vi "Take Outline Image.vi"(5 "Outline Width":dbl, 6 "Image Name":string="composite image", 7 "Quality":enum16{"perfect", "high", "medium", "low"}(ring), 8 "error in":errorcluster, 9 "Field of View":cluster{"Size-X(mm)":dbl, "Size-Y(mm)":dbl}, 10 "Image Center":refnum<class "Vec3d Class.lvclass">, 11 "CameraTool in":refnum<class "CameraTool Class.lvclass">) -> (0 "error out":errorcluster, 2 "Physical Image":T1, 3 "CameraTool out":refnum<class "CameraTool Class.lvclass">)   [LabVIEW 2017, in "CameraTool Class.lvclass"]
uses:
  CameraTool Class.lvclass
  Vec3d Class/Vec3d Class.lvclass
  <vilib>/vision/Image Controls.llb/IMAQ Image.ctl
  Utils/Type Definitions/Physical Image.ctl
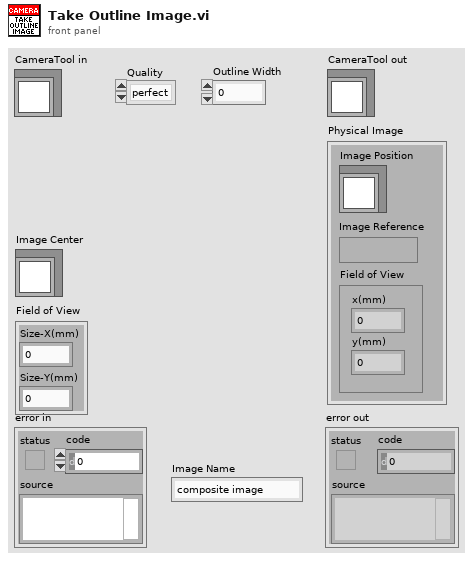
[diagram p1: front panel]
types:
  T1 = typedef "Physical Image.ctl" = cluster{"Image Position":refnum<class "Vec3d Class.lvclass">, "Image Reference":T2, "Field of View":cluster{"x(mm)":dbl, "y(mm)":dbl}}
  T2 = typedef "IMAQ Image.ctl" = refnum<image>
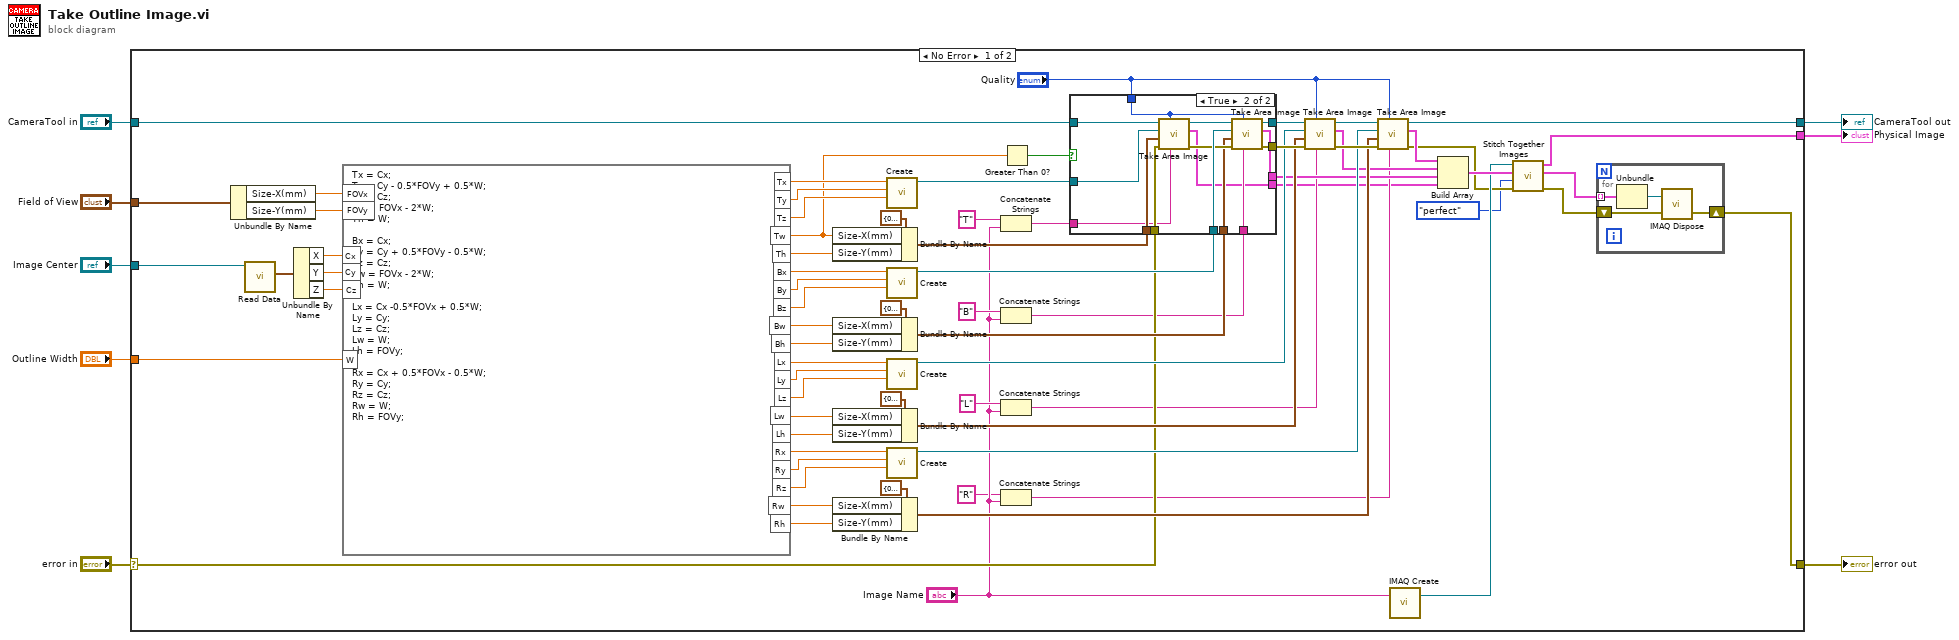
[diagram p0: block diagram]
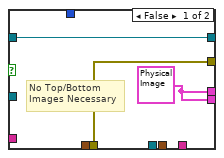
[diagram p2: hidden frame]
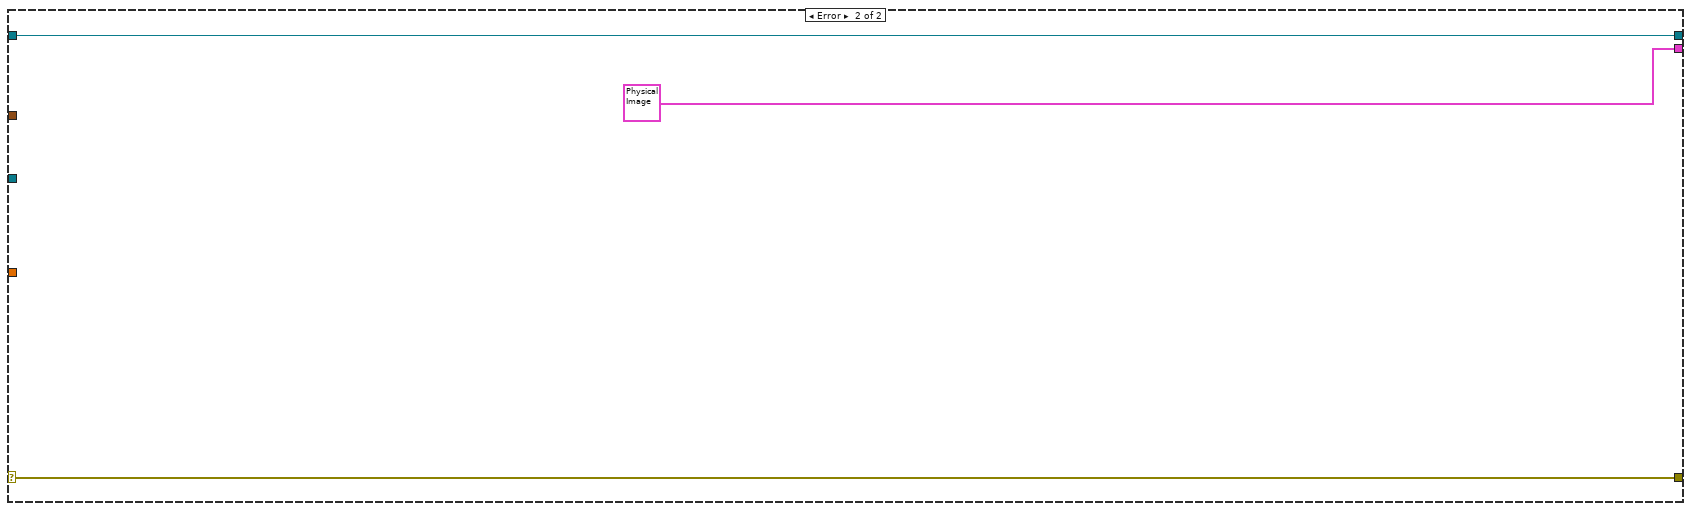
[diagram p3: hidden frame]
diagram:
  n1 = case shown="No Error" "error in" {
    selector: "error in" -> [w33 w104]
    tunnel: [w14 w104] -> w7
    tunnel: [w44 w103] -> w5
    tunnel: "CameraTool in" -> [w47 w103]
    tunnel: "Field of View" -> [w78 _]
    tunnel: "Image Center" -> [w79 _]
    tunnel: [w26 T1 {"Image Position"=refnum, "Image Reference"=refnum, "Field of View"={"x(mm)"=0.0, "y(mm)"=0.0}} ("Physical Image")] -> w2
    tunnel: "Outline Width" -> [w71 _]
    frame No Error {
      n2 = Unbundle By Name(w78) -> ("Size-X(mm)"=w77:dbl, "Size-Y(mm)"=w76:dbl)
      n3 = call-dynamic "Read Data.vi"("Vec3d Class in"=w79) -> ("Data"=w75:cluster{"X":dbl, "Y":dbl, "Z":dbl})  [unwired: 8 in, 2 out]
      n4 = Unbundle By Name(w75) -> ("X"=w74:dbl, "Y"=w73:dbl, "Z"=w72:dbl)
      n5 = formula code="Tx = Cx;\nTy = Cy - 0.5*FOVy + 0.5*W;\nTz = Cz;\nTw = FOVx - 2*W;\nTh = W;\n\nBx = Cx;\nBy = Cy + 0.5*FOVy - 0.5*W;\nBz = Cz;\nBw = FOVx - 2*W;\nBh = W;\n\nLx = Cx -0.5*FOVx + 0.5*W;\nLy = Cy;\nLz = Cz;\nLw = W;\nLh = FOVy;\n\nRx = Cx + 0.5*FOVx - 0.5*W;\nRy = Cy;\nRz = Cz;\nRw = W;\nRh = FOVy;"("Cx"=w74, "Cy"=w73, "Cz"=w72, "FOVx"=w77, "FOVy"=w76, "W"=w71) -> ("Tx"=w70:dbl, "Ty"=w69:dbl, "Tz"=w68:dbl, "Tw"=w12:dbl, "Th"=w66:dbl, "Bx"=w64:dbl, "By"=w63:dbl, "Bz"=w62:dbl, "Bw"=w61:dbl, "Bh"=w60:dbl, "Lx"=w58:dbl, "Ly"=w57:dbl, "Lz"=w56:dbl, "Lw"=w55:dbl, "Lh"=w54:dbl, "Rx"=w52:dbl, "Ry"=w51:dbl, "Rz"=w50:dbl, "Rw"=w49:dbl, "Rh"=w48:dbl)
      n6 = Bundle By Name(cluster=cluster{"Size-X(mm)":dbl, "Size-Y(mm)":dbl} {"Size-X(mm)"=0.0, "Size-Y(mm)"=0.0} ("Field of View"), "Size-X(mm)"=w12, "Size-Y(mm)"=w66) -> (w42:cluster{"Size-X(mm)":dbl, "Size-Y(mm)":dbl})
      n7 = Bundle By Name(cluster=cluster{"Size-X(mm)":dbl, "Size-Y(mm)":dbl} {"Size-X(mm)"=0.0, "Size-Y(mm)"=0.0} ("Field of View"), "Size-X(mm)"=w61, "Size-Y(mm)"=w60) -> (w38:cluster{"Size-X(mm)":dbl, "Size-Y(mm)":dbl})
      n8 = Bundle By Name(cluster=cluster{"Size-X(mm)":dbl, "Size-Y(mm)":dbl} {"Size-X(mm)"=0.0, "Size-Y(mm)"=0.0} ("Field of View"), "Size-X(mm)"=w55, "Size-Y(mm)"=w54) -> (w36:cluster{"Size-X(mm)":dbl, "Size-Y(mm)":dbl})
      n9 = Bundle By Name(cluster=cluster{"Size-X(mm)":dbl, "Size-Y(mm)":dbl} {"Size-X(mm)"=0.0, "Size-Y(mm)"=0.0} ("Field of View"), "Size-X(mm)"=w49, "Size-Y(mm)"=w48) -> (w34:cluster{"Size-X(mm)":dbl, "Size-Y(mm)":dbl})
      n10 = call "Create.vi"("Z"=w68, "Y"=w69, "X"=w70) -> ("Vec3d Class out"=w43:refnum<class "Vec3d Class.lvclass">)  [unwired: 7 in, 1 out]
      n11 = call "Create.vi"("Z"=w62, "Y"=w63, "X"=w64) -> ("Vec3d Class out"=w41:refnum<class "Vec3d Class.lvclass">)  [unwired: 7 in, 1 out]
      n12 = call "Create.vi"("Z"=w56, "Y"=w57, "X"=w58) -> ("Vec3d Class out"=w37:refnum<class "Vec3d Class.lvclass">)  [unwired: 7 in, 1 out]
      n13 = call "Create.vi"("Z"=w50, "Y"=w51, "X"=w52) -> ("Vec3d Class out"=w35:refnum<class "Vec3d Class.lvclass">)  [unwired: 7 in, 1 out]
      n14 = Concatenate Strings("T", "Image Name") -> (w24:string)
      n15 = Concatenate Strings("B", "Image Name") -> (w19:string)
      n16 = Concatenate Strings("L", "Image Name") -> (w18:string)
      n17 = Concatenate Strings("R", "Image Name") -> (w17:string)
      n18 = Greater Than 0?(x=w12) -> (x > 0?=w11:bool)
      n19 = case shown="True" w11 {
        tunnel: w47 -> [w86 w101]
        tunnel: [w86 w99] -> w46
        tunnel: "Quality" -> [_ w87]
        tunnel: w43 -> [_ w98]
        tunnel: w42 -> [_ w97]
        tunnel: w41 -> [_ w96]
        tunnel: [w84 w94] -> w40
        tunnel: w38 -> [_ w93]
        tunnel: w33 -> [w84 w92]
        tunnel: [w85 w91] -> w32
        tunnel: w24 -> [_ w90]
        tunnel: w19 -> [_ w89]
        tunnel: [w85 w88] -> w13
        frame False {
          w85 = T1 {"Image Position"=refnum, "Image Reference"=refnum, "Field of View"={"x(mm)"=0.0, "y(mm)"=0.0}} ("Physical Image")
          # "No Top/Bottom\nImages Necessary"
        }
        frame True {
          n20 = call "Take Area Image.vi"("Image Name"=w90, "Quality"=w87, "error in"=w92, "Field of View"=w97, "Image Center"=w98, "CameraTool in"=w101) -> ("error out"=w95:errorcluster, "Physical Image"=w88:T1, "CameraTool out"=w100:refnum<class "CameraTool Class.lvclass">)  [unwired: 3 in]
          n21 = call "Take Area Image.vi"("Image Name"=w89, "Quality"=w87, "error in"=w95, "Field of View"=w93, "Image Center"=w96, "CameraTool in"=w100) -> ("error out"=w94:errorcluster, "Physical Image"=w91:T1, "CameraTool out"=w99:refnum<class "CameraTool Class.lvclass">)  [unwired: 3 in]
        }
      }
      n22 = call "Take Area Image.vi"("Image Name"=w18, "Quality"="Quality", "error in"=w40, "Field of View"=w36, "Image Center"=w37, "CameraTool in"=w46) -> ("error out"=w39:errorcluster, "Physical Image"=w31:T1, "CameraTool out"=w45:refnum<class "CameraTool Class.lvclass">)  [unwired: 3 in]
      n23 = call "Take Area Image.vi"("Image Name"=w17, "Quality"="Quality", "error in"=w39, "Field of View"=w34, "Image Center"=w35, "CameraTool in"=w45) -> ("error out"=w27:errorcluster, "Physical Image"=w30:T1, "CameraTool out"=w44:refnum<class "CameraTool Class.lvclass">)  [unwired: 3 in]
      n24 = call "IMAQ Create"("Image Name"="Image Name") -> ("New Image"=w28:T2)  [unwired: 4 in, 1 out]
      n25 = Build Array(w30, w31, w32, w13) -> (w29:T1[])
      n26 = call "Stitch Together Images.vi"("error in"=w27, "Quality"=enum16{"perfect", "high", "medium", "low"}."perfect", "Physical Images in"=w29, "Image Dst"=w28) -> ("error out"=w15:errorcluster, "Physical Images out"=w16:T1[], "Composite Physical Image"=w26:T1)  [unwired: 5 in]
      n27 = for {
        tunnel: w16 -> [w83] mode=indexing
        shift-right: [w80] -> w14
        shift-left: w15 -> [w81]
        n28 = Unbundle(w83) -> ("Image Reference"=w82:T2)  [unwired: 2 out]
        n29 = call "IMAQ Dispose"("Image"=w82, "error in (no error)"=w81) -> ("error out"=w80:errorcluster)  [unwired: 4 in]
      }
    }
    frame Error {
    }
  }
  "error out" <- w7
  "CameraTool out" <- w5
  "Physical Image" <- w2
